vi "read_udc_float.vi"(1 "Hex Address":u16 format="%x") -> (0 "Value":dbl)   [LabVIEW 2011]
uses:
  <vilib>/NI Modbus.llb/MB Ethernet Master Query Read Input Registers (poly).vi
panel:
  out "Error Out":errorcluster
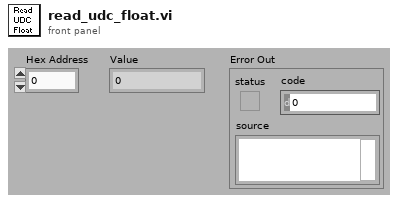
[diagram p1: front panel]
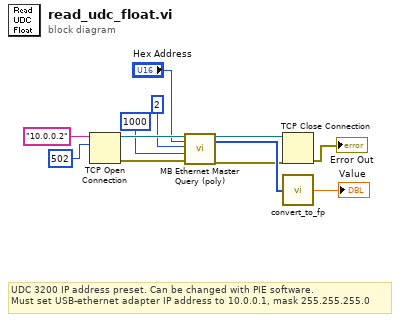
[diagram p0: block diagram]
diagram:
  # "UDC 3200 IP address preset. Can be changed with PIE software. \nMust set USB-ethernet adapter IP address to 10.0.0.1, mask 255.255.255.0"
  n1 = TCP Open Connection(address="10.0.0.2", remote port or service name=u16 502) -> (connection ID=w10:refnum<k5>, error out=w4:errorcluster)  [unwired: 1 in, 2 out]
  n2 = call-poly <vilib>:"MB Ethernet Master Query (poly).vi"("TCP Connection Refnum in"=w10, "Starting Address"="Hex Address", "Quantity"=u16 2, "Timeout"=1000, "error in"=w4) -> ("TCP Connection Refnum (dup)"=w9:refnum<k5>, "Input Registers"=w7:u16[], "error out"=w3:errorcluster)  [unwired: 12 out]
  n3 = TCP Close Connection(connection ID=w9, error in (no error)=w3) -> (error out=→"Error Out":errorcluster)  [unwired: 2 out]
  n4 = call "convert_to_fp.vi"("Input Array"=w7) -> ("Floating point"=→"Value":sgl)
